vi "H5Screate_simple.vi"(5 "max_dims":u64[](array[numeric]), 6 "dims":u64[](array[numeric]), 7 "error in (no error)":errorcluster) -> (0 "error out":errorcluster, 4 "space_id":i32)   [LabVIEW 2009]
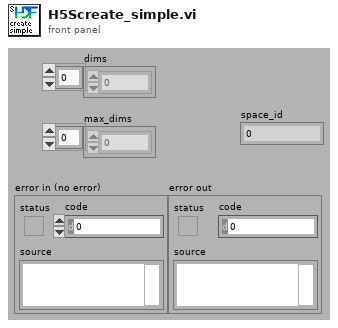
[diagram p1: front panel]
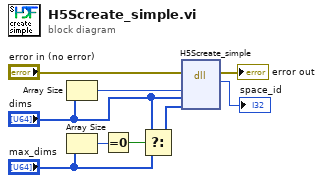
[diagram p0: block diagram]
diagram:
  n1 = Array Size(array="dims") -> (size(s)=w6:i32)
  n2 = Array Size(array="max_dims") -> (size(s)=w5:i32)
  n3 = Equal To 0?(x=w5) -> (x = 0?=w4:bool)
  n4 = Select(t="dims", s=w4, f="max_dims") -> (s? t:f=w1:u64[])
  n5 = dll-call lib="hdf5dll" fn="H5Screate_simple"(error in="error in (no error)", "rank"=w6, "dims"="dims", "max_dims"=w1) -> (error out=→"error out":errorcluster, "return type"=→"space_id":i32)  [unwired: 5 in, 1 out]
